vi "Accelerator GEMM And Operations.vi"(9 "Sessions Parameters":T3 {"graph_optimization_level" items=["ORT_DISABLE_ALL"=0, "ORT_ENABLE_ALL"=1, "ORT_ENABLE_BASIC"=2, "ORT_ENABLE_EXTENDED"=99]}, 10 "Execution Device":T1=enum."TensorRT", 11 "dimension size":i32=16384) -> (3 "Accelerator Time":dbl=0.19947869999998602)   [LabVIEW 2020]
uses:
  Source/Layer/Node/Gemm/_Controls/acc_gemm_param.ctl
  Source/_Controls/acc_execution_provider_enum.ctl
  Source/Model/Controls/acc_input_parameters.ctl
  Source/Layer/Node/_Controls/acc_onnx_dtype_enum.ctl
  Source/ONNX/_Controls/acc_tensorRT_ep_params_simplified.ctl
  Source/ONNX/Inference/acc_Inference.lvclass/acc_Inference.ctl
  Source/ONNX/Inference/_Methods/Simplified/acc_embedded_run_preallocated_multi_input_and_outputs_gpu_by_idx.vi
  Source/ONNX/Inference/_Methods/Simplified/acc_embedded_copy_ptr_data_to_labview_data.vi
  Source/ONNX/Inference/_Methods/Simplified/acc_embedded_run_mono_output_scalar_float.vi
  Source/SubVIs/sort_array/acc_sort_1d_index_ptr_data_cluster_array.vi
  Source/ONNX/Inference/_Methods/acc_embedded_run_preallocated_inputs_outputs_cuda_store_local.vi
  Source/SubVIs/sort_array/acc_sort_1d_index_out_ptr_data_cluster_array.vi
  Source/SubVIs/CUDAFunctions/acc_cuda_memcpy_device_to_host_bytes.vi
  Source/SubVIs/CUDAFunctions/acc_cuda_check_error.vi
  Source/SubVIs/CUDAFunctions/acc_cuda_error.vi
  Source/ONNX/Inference/acc_Inference.lvclass
  C:/Users/COCO/TDF Dropbox/1_Graiphic/3 - Services et Etudes/2 - Dev/code/Toolkits/Accelerator/Source/ONNX/acc_ONNX.lvclass
  Source/SubVIs/add_to_cluster_onnx_input/acc_onnx_add_scalar_float_array_into_ptr_input_cluster_array_by_idx.vi
  Source/SubVIs/add_to_cluster_onnx_input/acc_onnx_add_2d_float_array_into_ptr_input_cluster_array_by_idx.vi
  Source/Model/_Methods/add_to_graph/Initializer/acc_float_scalar_initializer.vi
  Source/Model/_Methods/add_to_graph/Numeric/acc_add_adaptive.vi
  Source/Model/_Methods/acc_create_onnx_model_then_init_cuda_inference_session.vi
  Source/Model/_Methods/acc_create_onnx_model_then_init_inference_session.vi
  Source/Model/_Methods/acc_create_onnx_model_then_init_tensorRT_inference_session.vi
  Source/ONNX/Inference/_Methods/acc_embedded_check_execution_inputs_index.vi
  Source/ONNX/Inference/_Methods/acc_embedded_check_execution_outputs_index.vi
  Source/ONNX/_Accessors/acc_Read dll_path.vi
  Source/ONNX/SubVIs/acc_ONNX_CheckError.vi
  Source/SubVIs/CUDAFunctions/cuda_path_without_check_version.vi
  Source/SubVIs/Acc_ErrorStop.vi
  Source/SubVIs/checks/acc_check_output_onnx.vi
  Source/Model/acc_Model.lvclass
  <vilib>/Analysis/NI_AALBase.lvlib
panel:
  in  "Parameters":T2={"alpha"=1.0, "beta"=0.0, "transA"=0, "transB"=0}
  out "max value":sgl=5.4420166
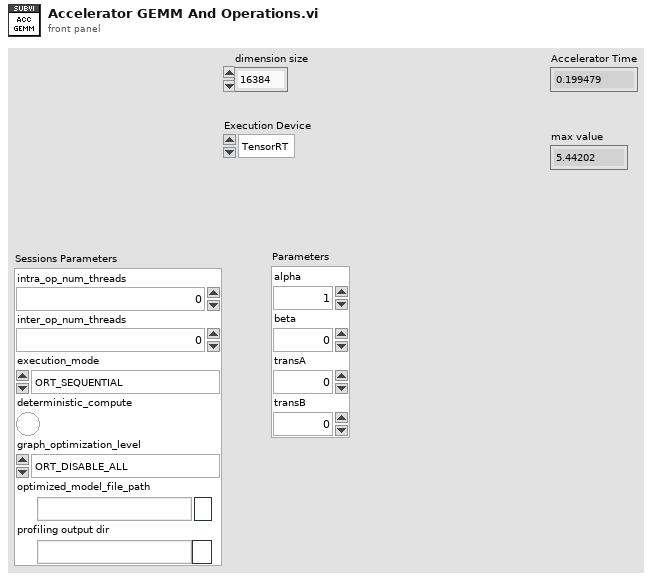
[diagram p1: front panel]
types:
  T1 = typedef "acc_execution_provider_enum.ctl" = enum16{"CPU", "CUDA", "TensorRT"}
  T2 = typedef "acc_gemm_param.ctl" = cluster{"alpha":sgl, "beta":sgl, "transA":i64, "transB":i64}
  T3 = cluster{"intra_op_num_threads":i32, "inter_op_num_threads":i32, "execution_mode":enum16{"ORT_SEQUENTIAL", "ORT_PARALLEL"}, "deterministic_compute":bool, "graph_optimization_level":u16, "optimized_model_file_path":path, "profiling output dir":path}
  T4 = typedef "acc_input_parameters.ctl" = cluster{"Rank":enum16{"Scalar", "1D", "2D", "3D", "4D", "5D", "6D"}, "dtype":T5, "complex?":bool, "expert?":bool}
  T5 = typedef "acc_onnx_dtype_enum.ctl" = enum16{"UNDEFINED", "FLOAT", "UINT8", "INT8", "UINT16", "INT16", "INT32", "INT64", "STRING", "BOOL", "FLOAT16", "DOUBLE", "UINT32", "UINT64", "COMPLEX64", "COMPLEX128", "BFLOAT16", "FLOAT8E4M3FN", "FLOAT8E4M3FNUZ", "FLOAT8E5M2", "FLOAT8E5M2FNUZ", "UINT4", "INT4"}
  T6 = typedef "acc_onnx_multi_ptr_input_index_cluster.ctl" = cluster{"input_order":u32, "Inputs Info":cluster{"inputs_ptr":u64, "inputs_shapes":i64[], "inputs_ranks":i64, "inputs_types":T5}}
  T7 = typedef "acc_tensorRT_ep_params_simplified.ctl" = cluster{"Device And Stream":cluster{"Device Index":i32, "Use Custom Compute Stream?":bool, "Custom Compute Stream (Pointer)":u64}, "Parser & Subgraph Options":cluster{"Max Partition Attemps":i32, "Minimum Subgraph Size":i32}, "Memory & Workspace Management":cluster{"Max Workspace Memory (Bytes)":u64, "Share Memory Between Subgraphs":bool, "Auxiliary Stream Count":i32}, "Precision & Numeric Modes":cluster{"Enable FP16":bool, "Enable BF16":bool, "Enable INT8":bool, "INT8 Calibration Table Name":path, "Use Native INT8 Calibration?":bool}, "Engine Build, Cache & Paths":cluster{"Enable Engine Caching?":bool, "Engine Cache Directory":path, "Enable Engine Decryption?":bool, "Decryption Library Path":path, "Build Engines Sequentially?":bool, "Enable Timing Cache?":bool, "Timing Cache Directory":path, "Force Timing Cache Use?":bool, "Enable Detailed Logs?":bool, "Use Build Heuristics?":bool, "Enable Weight Sparsity?":bool, "Engine Optimization Level (0–5)":i32}, "Paths & Plugins":cluster{"Extra Plugin Libraries":path[], "Tactic Source Rules":string, "Enabled Preview Features":enum16{"None", "ALIASED_PLUGIN_IO_10_03"}}, "Profile Shapes":cluster{"Minimum Input Shapes":string, "Maximum Input Shapes":string, "Optimal Input Shapes":string}, "Advanced & DLA / CUDA Graph":cluster{"Enable DLA Acceleration?":bool, "DLA Core Index":i32, "Dump TensorRT Subgraphs?":bool, "Force LayerNorm in FP32?":bool, "Enable CUDA Graph Execution?":bool}}
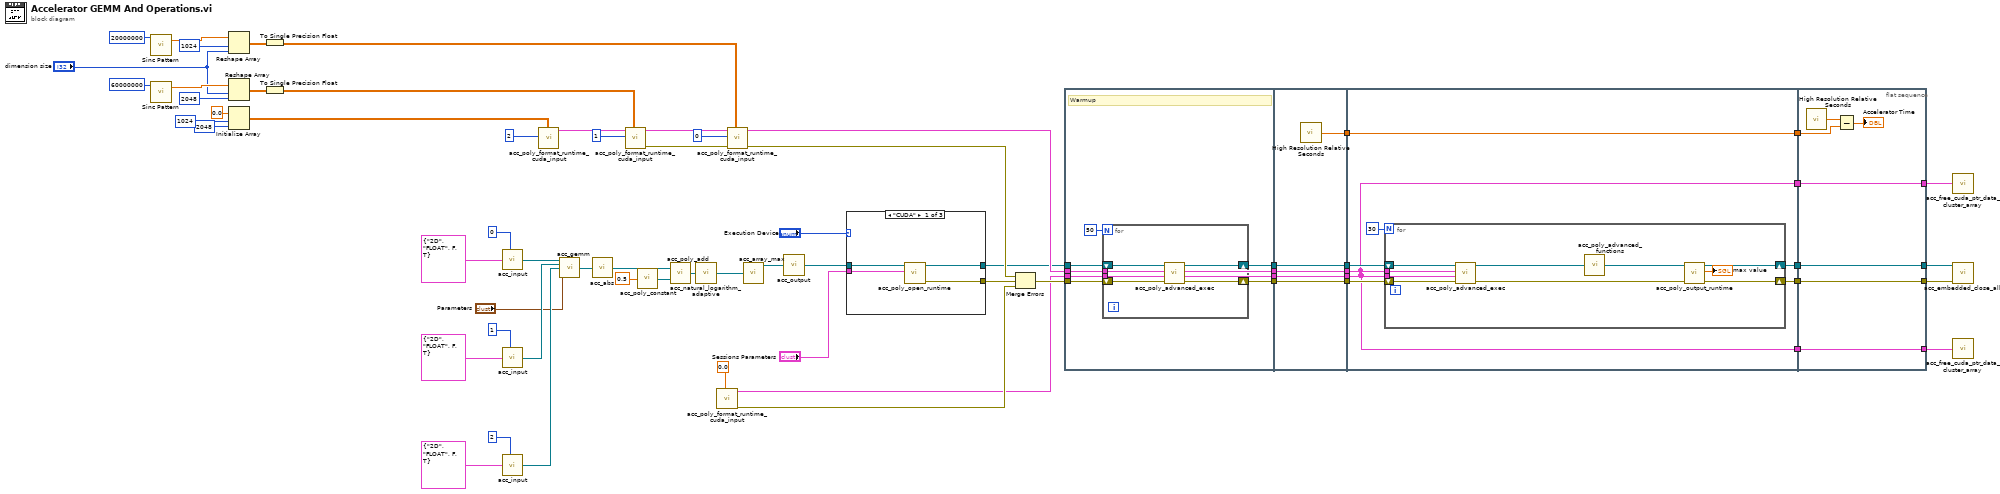
[diagram p0: block diagram]
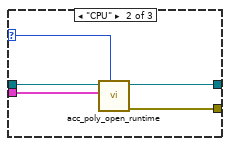
[diagram p2: hidden frame]
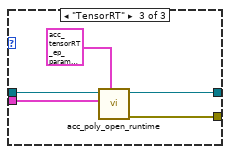
[diagram p3: hidden frame]
diagram:
  n1 = call <vilib>:"Sinc Pattern.vi"("samples"=20000000) -> ("Sinc Pattern"=w61:dbl[])  [unwired: 3 in, 1 out]
  n2 = call <vilib>:"Sinc Pattern.vi"("samples"=60000000) -> ("Sinc Pattern"=w60:dbl[])  [unwired: 3 in, 1 out]
  n3 = Reshape Array(w61, 1024 ("dimension size"), "dimension size") -> (w55:dbl[][])
  n4 = Reshape Array(w60, "dimension size", 2048 ("dimension size")) -> (w54:dbl[][])
  n5 = Initialize Array(sgl 0.0 ("element"), 1024 ("dimension size"), 2048 ("dimension size")) -> (w12:sgl[][])
  n6 = To Single Precision Float(number=w55) -> (single precision float=w13:sgl[][])
  n7 = To Single Precision Float(number=w54) -> (single precision float=w11:sgl[][])
  n8 = call "acc_input.vi"("index"=0, "Parameters"=T4 {"Rank"=enum."2D", "dtype"=enum."FLOAT", "complex?"=FALSE, "expert?"=TRUE}) -> ("ONNXModel out"=w29:refnum<class "acc_Model.lvclass">)  [unwired: 7 in]
  n9 = call "acc_input.vi"("index"=1, "Parameters"=T4 {"Rank"=enum."2D", "dtype"=enum."FLOAT", "complex?"=FALSE, "expert?"=TRUE}) -> ("ONNXModel out"=w28:refnum<class "acc_Model.lvclass">)  [unwired: 7 in]
  n10 = call "acc_input.vi"("index"=2, "Parameters"=T4 {"Rank"=enum."2D", "dtype"=enum."FLOAT", "complex?"=FALSE, "expert?"=TRUE}) -> ("ONNXModel out"=w20:refnum<class "acc_Model.lvclass">)  [unwired: 7 in]
  n11 = call-poly "acc_poly_format_runtime_cuda_input.vi"("2D Input Data"=w12, "input order"=2) -> ("Data in"=w18:T6[])  [unwired: 8 in, 1 out]
  n12 = call "acc_gemm.vi"("A"=w29, "B"=w28, "C"=w20, "Parameters"="Parameters") -> ("subarray"=w27:refnum<class "acc_Model.lvclass">)  [unwired: 11 in]
  n13 = call "acc_abs.vi"("x"=w27) -> ("abs(x)"=w17:refnum<class "acc_Model.lvclass">)
  n14 = call-poly "acc_poly_format_runtime_cuda_input.vi"("2D Input Data"=w11, "input order"=1, "Data in"=w18) -> ("error out"=w46:errorcluster, "Data in"=w49:T6[])  [unwired: 7 in]
  n15 = call-poly "acc_poly_constant.vi"("scalar"=sgl 0.5) -> ("Float Scalar"=w15:refnum<class "acc_Model.lvclass">)  [unwired: 3 in]
  n16 = call-poly "acc_poly_add.vi"("y"=w15, "x"=w17) -> ("x+y"=w14:refnum<class "acc_Model.lvclass">)
  n17 = call "acc_natural_logarithm_adaptive.vi"("x"=w14) -> ("ln(x)"=w34:refnum<class "acc_Model.lvclass">)
  n18 = call-poly "acc_poly_format_runtime_cuda_input.vi"("Input Data"=sgl 0.0) -> ("error out"=w44:errorcluster, "Data in"=w9:T6[])  [unwired: 9 in]
  n19 = call-poly "acc_poly_format_runtime_cuda_input.vi"("2D Input Data"=w13, "error in"=w46, "input order"=0, "Data in"=w49) -> ("error out"=w45:errorcluster, "Data in"=w8:T6[])  [unwired: 6 in]
  n20 = call "acc_array_max.vi"("array"=w34) -> ("max value"=w57:refnum<class "acc_Model.lvclass">)  [unwired: 6 in, 1 out]
  n21 = call "acc_output.vi"("ONNXModel in"=w57) -> ("ONNXModel out"=w5:refnum<class "acc_Model.lvclass">)  [unwired: 8 in]
  n22 = case shown="\"CUDA\"" "Execution Device" {
    selector: "Execution Device" -> [_ w72 _]
    tunnel: [w71 w76 w81] -> w4
    tunnel: [w70 w75 w80] -> w3
    tunnel: "Sessions Parameters" -> [w69 w74 w79]
    tunnel: w5 -> [w68 w73 w78]
    frame "CUDA" {
      n23 = call-poly "acc_poly_open_runtime.vi"("Sessions Parameters"=w69, "Model in"=w68) -> ("error out"=w70:errorcluster, "Inference out"=w71:refnum<class "acc_Inference.lvclass">)  [unwired: 8 in]
    }
    frame "CPU" {
      n24 = call-poly "acc_poly_open_runtime.vi"("Execution Device"=w72, "Sessions Parameters"=w74, "Model in"=w73) -> ("error out"=w75:errorcluster, "Inference out"=w76:refnum<class "acc_Inference.lvclass">)  [unwired: 7 in]
    }
    frame "TensorRT" {
      n25 = call-poly "acc_poly_open_runtime.vi"("TRT Parameters"=T7 {"Device And Stream"={"Device Index"=0, "Use Custom Compute Stream?"=FALSE, "Custom Compute Stream (Pointer)"=0}, "Parser & Subgraph Options"={"Max Partition Attemps"=1000, "Minimum Subgraph Size"=1}, "Memory & Workspace Management"={"Max Workspace Memory (Bytes)"=0, "Share Memory Between Subgraphs"=FALSE, "Auxiliary Stream Count"=-1}, "Precision & Numeric Modes"={"Enable FP16"=FALSE, "Enable BF16"=FALSE, "Enable INT8"=FALSE, "INT8 Calibration Table Name"=path "", "Use Native INT8 Calibration?"=FALSE}, "Engine Build, Cache & Paths"={"Enable Engine Caching?"=FALSE, "Engine Cache Directory"=path "", "Enable Engine Decryption?"=FALSE, "Decryption Library Path"=path "", "Build Engines Sequentially?"=FALSE, "Enable Timing Cache?"=FALSE, "Timing Cache Directory"=path "", "Force Timing Cache Use?"=FALSE, "Enable Detailed Logs?"=FALSE, "Use Build Heuristics?"=FALSE, "Enable Weight Sparsity?"=FALSE, "Engine Optimization Level (0–5)"=3}, "Paths & Plugins"={"Extra Plugin Libraries"=[], "Tactic Source Rules"="", "Enabled Preview Features"=enum."None"}, "Profile Shapes"={"Minimum Input Shapes"="", "Maximum Input Shapes"="", "Optimal Input Shapes"=""}, "Advanced & DLA / CUDA Graph"={"Enable DLA Acceleration?"=FALSE, "DLA Core Index"=0, "Dump TensorRT Subgraphs?"=FALSE, "Force LayerNorm in FP32?"=FALSE, "Enable CUDA Graph Execution?"=FALSE}}, "Sessions Parameters"=w79, "Model in"=w78) -> ("error out"=w80:errorcluster, "Inference out"=w81:refnum<class "acc_Inference.lvclass">)  [unwired: 7 in]
    }
  }
  n26 = Merge Errors(w45, w3, w44) -> (w42:errorcluster)
  n27 = flat-sequence {
    tunnel: w42 -> [w86]
    tunnel: w8 -> [w85]
    tunnel: w9 -> [w84]
    tunnel: w4 -> [w88]
    tunnel: [w87] -> w33
    tunnel: [w85] -> w32
    tunnel: [w84] -> w31
    tunnel: [w83] -> w30
    tunnel: [w99] -> w65
    tunnel: [w98] -> w56
    tunnel: [w97] -> w48
    tunnel: [w96] -> w47
    tunnel: [w95] -> w43
    tunnel: w33 -> [w98]
    tunnel: w32 -> [w96]
    tunnel: w31 -> [w97]
    tunnel: w30 -> [w95]
    tunnel: w65 -> [w107]
    tunnel: [w107] -> w64
    tunnel: w56 -> [w105]
    tunnel: w48 -> [w100]
    tunnel: w47 -> [w101]
    tunnel: w43 -> [w104]
    tunnel: [w103] -> w40
    tunnel: [w102] -> w39
    tunnel: [w101] -> w37
    tunnel: [w100] -> w36
    tunnel: w64 -> [w123]
    tunnel: [w121] -> w41
    tunnel: w40 -> [w121]
    tunnel: w39 -> [w120]
    tunnel: [w120] -> w38
    tunnel: [w119] -> w7
    tunnel: w37 -> [w119]
    tunnel: [w118] -> w6
    tunnel: w36 -> [w118]
    frame #0 {
      # "Warmup"
      n28 = for {
        N: 50 -> [_]
        tunnel: w85 -> [w91]
        tunnel: w84 -> [w90]
        shift-right: [w93] -> w87
        shift-left: w88 -> [w94]
        shift-right: [w89] -> w83
        shift-left: w86 -> [w92]
        n29 = call-poly "acc_poly_advanced_exec.vi"("error in"=w92, "Data out"=w90, "Data in"=w91, "Inference in"=w94) -> ("error out"=w89:errorcluster, "Inference out"=w93:refnum<class "acc_Inference.lvclass">)  [unwired: 6 in]
      }
    }
    frame #1 {
      n30 = call <vilib>:"High Resolution Relative Seconds.vi"() -> ("relative seconds"=w99:dbl)
    }
    frame #2 {
      n31 = for {
        N: 30 -> [_]
        tunnel: w100 -> [w116]
        tunnel: w101 -> [w115]
        shift-right: [w111] -> w103
        shift-left: w105 -> [w117]
        shift-right: [w110] -> w102
        shift-left: w104 -> [w114]
        n32 = call-poly "acc_poly_advanced_exec.vi"("error in"=w114, "Data out"=w116, "Data in"=w115, "Inference in"=w117) -> ("error out"=w112:errorcluster, "Inference out"=w113:refnum<class "acc_Inference.lvclass">)  [unwired: 6 in]
        n33 = call-poly "acc_poly_advanced_functions.vi"("Inference in"=w113) -> ("Inference out"=w109:refnum<class "acc_Inference.lvclass">)
        n34 = call-poly "acc_poly_output_runtime.vi"("error in"=w112, "Inference in"=w109) -> ("error out"=w110:errorcluster, "Output Data"=→"max value":sgl, "Inference out"=w111:refnum<class "acc_Inference.lvclass">)  [unwired: 7 in]
      }
    }
    frame #3 {
      n35 = call <vilib>:"High Resolution Relative Seconds.vi"() -> ("relative seconds"=w124:dbl)
      n36 = Subtract(x=w124, y=w123) -> (x-y=→"Accelerator Time":dbl)
    }
  }
  n37 = call "acc_free_cuda_ptr_data_cluster_array.vi"("Data in"=w7) -> ()
  n38 = call-dynamic "acc_embedded_close_all.vi"("error in"=w38, "Inference in"=w41) -> ()  [unwired: 8 in, 2 out]
  n39 = call "acc_free_cuda_ptr_data_cluster_array.vi"("Data in"=w6) -> ()
